vi "about get number of organized files.vi"(8 "error in (no error)":errorcluster) -> (0 "error out":errorcluster, 3 "Number of Organized Files":i32)   [LabVIEW 2011]
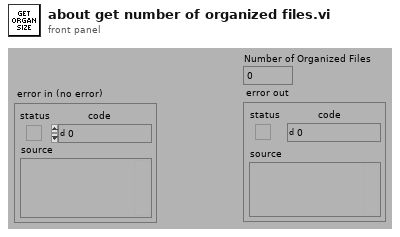
[diagram p1: front panel]
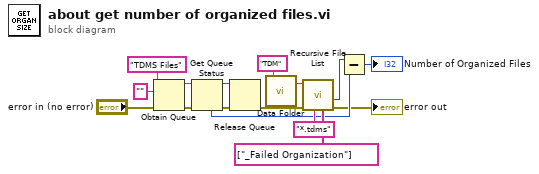
[diagram p0: block diagram]
diagram:
  n1 = Obtain Queue(name (unnamed)="TDMS Files", element data type="", error in (no error)="error in (no error)") -> (queue out=w9:refnum<queue>, error out=w12:errorcluster)  [unwired: 2 in, 1 out]
  n2 = Get Queue Status(queue=w9, error in (no error)=w12) -> (queue out=w10:refnum<queue>, error out=w11:errorcluster, # elements in queue=w4:i32)  [unwired: 1 in, 5 out]
  n3 = Release Queue(queue=w10, error in (no error)=w11) -> (error out=w8:errorcluster)  [unwired: 1 in, 2 out]
  n4 = call "Data Folder.vi"("Relative Path (\"\" - Folder)"="TDM" ("Relative Path (\"\" - Folder)")) -> ("Data Folder"=w15:path)  [unwired: 2 in]
  n5 = call <vilib>:"Recursive File List.vi"("Folders to Exclude"=string[] ["_Failed Organization"], "pattern"="*.tdms", "error in (no error)"=w8, "Folder Path"=w15) -> ("error out"=→"error out":errorcluster, "Number of Files"=w5:i32)  [unwired: 3 in, 3 out]
  n6 = Subtract(x=w5, y=w4) -> (x-y=→"Number of Organized Files":i32)
